vi "MT Generate Bits (Fibonacci, Primitive Polynomial).vi"(0 "total bits (128)":i32=128, 7 "specify primitive polynomial":i8[](array[numeric]), 9 "seed in (0xD6BF7DF2)":i32=169 format="%.0b", 11 "error in (no error)":errorcluster, 13 "reset? (T)":bool=TRUE) -> (4 "output bit stream":i8[](array[numeric]), 10 "seed out":i32 format="%.0x", 15 "error out":errorcluster)   [LabVIEW 2020, in "niDMT.lvlib"]
doc: "This polymorphic instance generates Fibonacci pseudonoise (PN) bit sequences. The VI repeats the selected pattern until it generates number of total bits that you specify. Use this instance to specify the primitive polynomial that determines the connection structure of the linear feedback shift register (LFSR)."
uses:
  <vilib>/addons/Modulation/niDMT.lvlib
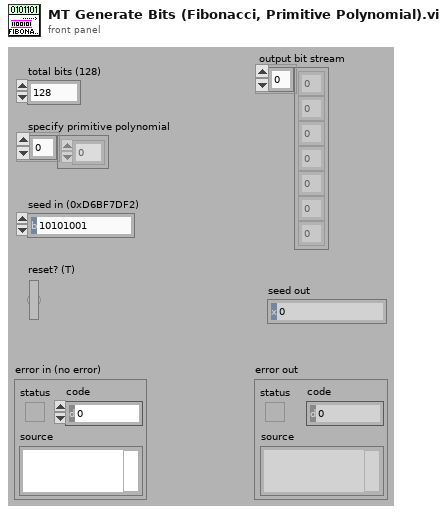
[diagram p1: front panel]
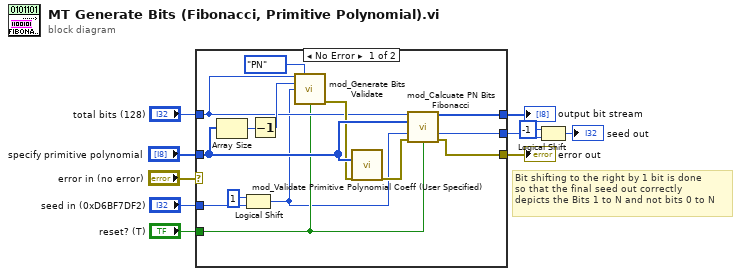
[diagram p0: block diagram]
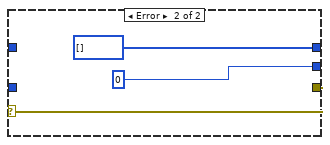
[diagram p2: hidden frame]
diagram:
  # "Bit shifting to the right by 1 bit is done \nso that the final seed out correctly \ndepicts the Bits 1 to N and not bits 0 to N"
  n1 = case shown="No Error" "error in (no error)" {
    selector: "error in (no error)" -> [_ w27]
    tunnel: "seed in (0xD6BF7DF2)" -> [w12 _]
    tunnel: "total bits (128)" -> [w16 _]
    tunnel: [w19 i8[] []] -> w8
    tunnel: [w21 w27] -> w6
    tunnel: [w20 0] -> w2
    tunnel: "reset? (T)" -> [w14 _]
    tunnel: "specify primitive polynomial" -> [w23 _]
    frame No Error {
      n2 = Array Size(array=w23) -> (size(s)=w24:i32)
      n3 = Logical Shift(y=1, x=w12) -> (x << y=w11:i32)
      n4 = Decrement(x=w24) -> (x-1=w17:i32)
      n5 = call <vilib>:"mod_Generate Bits Validate.vi"("Total Bits"=w16, "Mode (PN)"=enum16{"PN", "pattern", "user"}."PN", "PN Sequence Order"=w17, "seed in"=w11, "reset?"=w14) -> ("error out"=w18:errorcluster)  [unwired: 2 in, 8 out]
      n6 = call <vilib>:"mod_Validate Primitive Polynomial Coeff (User Specified).vi"("specify primitive polynomial"=w23, "error in (no error)"=w18) -> ("error out"=w22:errorcluster)  [unwired: 1 in, 12 out]
      n7 = call <vilib>:"mod_Calcuate PN Bits Fibonacci.vi"("total bits (128)"=w16, "primitive polynomial"=w23, "seed in (0xD6BF7DF2)"=w11, "error in (no error)"=w22, "reset? (T)"=w14) -> ("output bits"=w19:i8[], "seed out"=w20:i32, "error out"=w21:errorcluster)  [unwired: 1 in, 7 out]
    }
    frame Error {
    }
  }
  "output bit stream" <- w8
  "error out" <- w6
  n8 = Logical Shift(y=-1, x=w2) -> (x << y=→"seed out":i32)
